vi "Update FOV-retd.vi"(8 "error in (no error)":errorcluster, 11 "UI ctrl refs":T1) -> (0 "error out":errorcluster)   [LabVIEW 2020]
uses:
  Typedefs/Plane Mode.ctl
  Typedefs/Laser control knob.ctl
  Typedefs/PMT control knob.ctl
  Typedefs/XY Stage_Move.ctl
  Typedefs/Frame Size.ctl
  Typedefs/UI ctrl refs cluster.ctl
  Acquisition/Typedefs/Ref DAQ Param.ctl
  Typedefs/test_fpga_control.ctl
  Biology Information.ctl
  Experiment Type.ctl
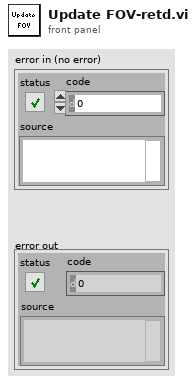
[diagram p1: front panel]
types:
  T1 = typedef "UI ctrl refs cluster.ctl" = cluster{"Top level VI path":path, "Top level VI ref":refnum<vi>, "User menu ref":refnum<k9>, "Sub Panel control":refnum<vi>, "Imaging Param Tab":refnum<vi>, "Occurrence-Start drivers":refnum<k4>, "Occurrence-Speed logging initialised":refnum<k4>, "Occurrence-XYZ stage initialised":refnum<k4>, "Exit button":refnum<vi>, "Status ind":refnum<vi>, "Set as origin":refnum<vi>, "Speed Logging":refnum<vi>, "Time Lapse":refnum<vi>, "Live Imaging":refnum<vi>, "AOL Z Stack":refnum<vi>, "Motor Z Stack":refnum<vi>, "Funct Acq button":refnum<vi>, "Hard Shutter":refnum<vi>, "Virtual Shutter":refnum<vi>, "Laser Power":refnum<vi>, "AOL Mode":refnum<vi>, "Frame Size":refnum<vi>, "Field of View":refnum<vi>, "Dwell Time":refnum<vi>, "Zoom":refnum<vi>, "AOL Z":refnum<vi>, "Objective":refnum<vi>, "Axis":refnum<vi>, "Paths & Names":refnum<vi>, "Experiment folder path (ind.)":refnum<vi>, "Last State (Ind.)":refnum<vi>, "Averages":refnum<vi>, "Angle (degrees)":refnum<vi>, "X centre":refnum<vi>, "Y centre":refnum<vi>, "Plane Mode":refnum<vi>, "# Planes":refnum<vi>, "Z Start":refnum<vi>, "Z Stop":refnum<vi>, "Z Step":refnum<vi>, "PMT 1":refnum<vi>, "PMT 2":refnum<vi>, "Stage XYZ Position":refnum<vi>, "Pockels@Z Start":refnum<vi>, "Pockels@Z Stop":refnum<vi>, "Obtain Z Start":refnum<vi>, "Obtain Z Stop":refnum<vi>, "Live stim.trig.period":refnum<vi>, "Live stim.trig.enable":refnum<vi>, "Movement Correction":refnum<vi>, "Load Reference Image":refnum<vi>, "XY Stage Move":refnum<vi>, "MovCor Cluster":refnum<vi>, "RefDAQParam":refnum<vi>, "Funct. Acq. Pockels Modulation":refnum<vi>, "Ref Laser Power":refnum<vi>, "Enable Video Recording":refnum<vi>, "Video Record-Live Imaging":refnum<vi>, "Video Record-Funct acq":refnum<vi>, "Reference Source":refnum<vi>, "AOL Z-stack Chirps Ready (ind)":refnum<vi>, "Target time between mov.cor. ref triggers (ms)":refnum<vi>, "Funct. Acq. Ref frame save":refnum<vi>, "Tracking button":refnum<vi>, "Show ref plots window":refnum<vi>, "Center freq ind (nm)":refnum<vi>, "Pickup mode (ind)":refnum<vi>, "Logging queue (ind)":refnum<vi>, "Back aperture power (ind.)":refnum<vi>, "Power after objective (ind.)":refnum<vi>, "Switch user":refnum<vi>, "Ls1 Conn. Status":refnum<vi>, "Ls1Tuning Status":refnum<vi>, "Ls1 Faults":refnum<vi>, "Ls1 Connection":refnum<vi>, "Ls1 Mode":refnum<vi>, "Ls1 POWER [mW]":refnum<vi>, "Ls1Shutter":refnum<vi>, "Ls1 Wavelength":refnum<vi>, "Ls1 Note":refnum<vi>, "Ls1 Confirm Wav":refnum<vi>, "Ls1 PreChrp Prism1":refnum<vi>, "Ls1 PreChrp Prism2":refnum<vi>, "Ls1 wav top Ind":refnum<vi>, "Ls1 power top Ind":refnum<vi>, "Ls1 Pump peak Hold":refnum<vi>, "Ls1 Status Ind":refnum<vi>, "Ls1 wav cancel":refnum<vi>, "Experiment Type":refnum<vi>, "Biology Information":refnum<vi>, "Camera recording status":refnum<vi>, "Optimise Obj. Pos.":refnum<vi>}
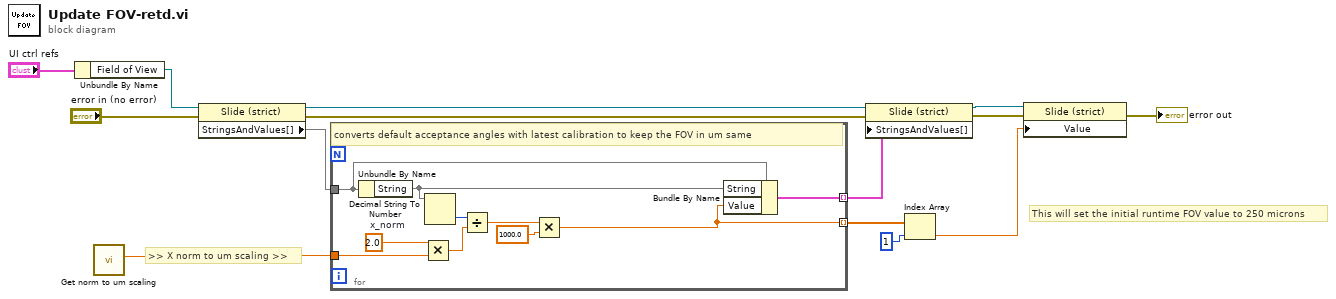
[diagram p0: block diagram]
diagram:
  # ">> X norm to um scaling >>"
  # "This will set the initial runtime FOV value to 250 microns"
  n1 = Unbundle By Name("UI ctrl refs") -> ("Field of View"=w14:refnum<vi>)
  n2 = call "Get norm to um scaling .vi"() -> ("X_norm to um_scaling"=w1:dbl)  [unwired: 8 in, 3 out]
  n3 = property on="Property Node" class="Slide (strict)"(reference=w14, error in="error in (no error)") -> (reference out=w8:refnum<vi>, error out=w11:errorcluster, "StringsAndValues[]"=w13)
  n4 = for {
    tunnel: w13 -> [w24]
    tunnel: [w23] -> w12 mode=indexing
    tunnel: w1 -> [w20]
    tunnel: [w15] -> w7 mode=indexing
    w21 = 2.0  # x_norm
    # "converts default acceptance angles with latest calibration to keep the FOV in um same"
    n5 = Unbundle By Name(w24) -> ("String"=w17)
    n6 = Multiply(x=w21, y=w20) -> (x*y=w22:dbl)
    n7 = Decimal String To Number(string=w17) -> (number=w16:i32)  [unwired: 2 in, 1 out]
    n8 = Divide(x=w16, y=w22) -> (x/y=w19:dbl)
    n9 = Multiply(x=w19, y=1000.0) -> (x*y=w15:dbl)
    n10 = Bundle By Name(cluster=w24, "String"=w17, "Value"=w15) -> (w23:cluster{})
  }
  n11 = property on="Property Node" class="Slide (strict)"(reference=w8, error in=w11, "StringsAndValues[]"=w12) -> (reference out=w3:refnum<vi>, error out=w2:errorcluster)
  n12 = Index Array(array=w7, index=1) -> (element=w6:dbl)
  n13 = property class="Slide (strict)"(reference=w3, error in=w2, "Value"=w6) -> (error out=→"error out":errorcluster)  [unwired: 1 out]
